vi "Update Library Icon.vi"(8 "error in (no error)":errorcluster, 11 "Mock Class Generator In":refnum<class "Responsive Mock Class Generator.lvclass">) -> (0 "error out":errorcluster, 3 "Mock Class Generator Out":refnum<class "Responsive Mock Class Generator.lvclass">)   [LabVIEW 2020, in "Responsive Mock Class Generator.lvclass"]
uses:
  Responsive Mock Class Generator.lvclass
  <vilib>/LabVIEW Icon API/lv_icon/Classes/Icon/Icon.lvclass
  <vilib>/LabVIEW Icon API/API_Rectangle Dimension.ctl
  <vilib>/LabVIEW Icon API/API_Text.ctl
  <vilib>/LabVIEW Icon API/API_Test Settings.ctl
  <vilib>/LabVIEW Icon API/lv_icon/Controls/Alignment.ctl
  <vilib>/LabVIEW Icon API/API_Text Colors.ctl
  <vilib>/LabVIEW Icon API/API_Rectangle Colors.ctl
  Responsive Mock Class Generator.lvclass/Responsive Mock Class Generator.ctl
  <vilib>/LabVIEW Icon API/LabVIEW Icon API.lvlib
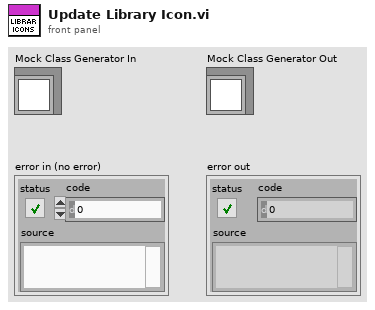
[diagram p1: front panel]
types:
  T1 = typedef "LabVIEW Icon API.lvlib/API_Rectangle Colors.ctl" = cluster{"Border":u32, "Background":u32}
  T2 = typedef "LabVIEW Icon API.lvlib/API_Test Settings.ctl" = cluster{"Font":string, "Alignment":T3, "Size":u8, "Center text":bool, "Capitalize text":bool, "Text color":T4}
  T3 = typedef "Alignment.ctl" = u16
  T4 = typedef "LabVIEW Icon API.lvlib/API_Text Colors.ctl" = cluster{"Line 1 color":u32, "Line 2 color":u32, "Line 3 color":u32, "Line 4 color":u32}
  T5 = typedef "LabVIEW Icon API.lvlib/API_Text.ctl" = cluster{"Line 1 text":string, "Line 2 text":string, "Line 3 text":string, "Line 4 text":string}
  T6 = typedef "LabVIEW Icon API.lvlib/API_Rectangle Dimension.ctl" = cluster{"Width":i16, "Height":i16}
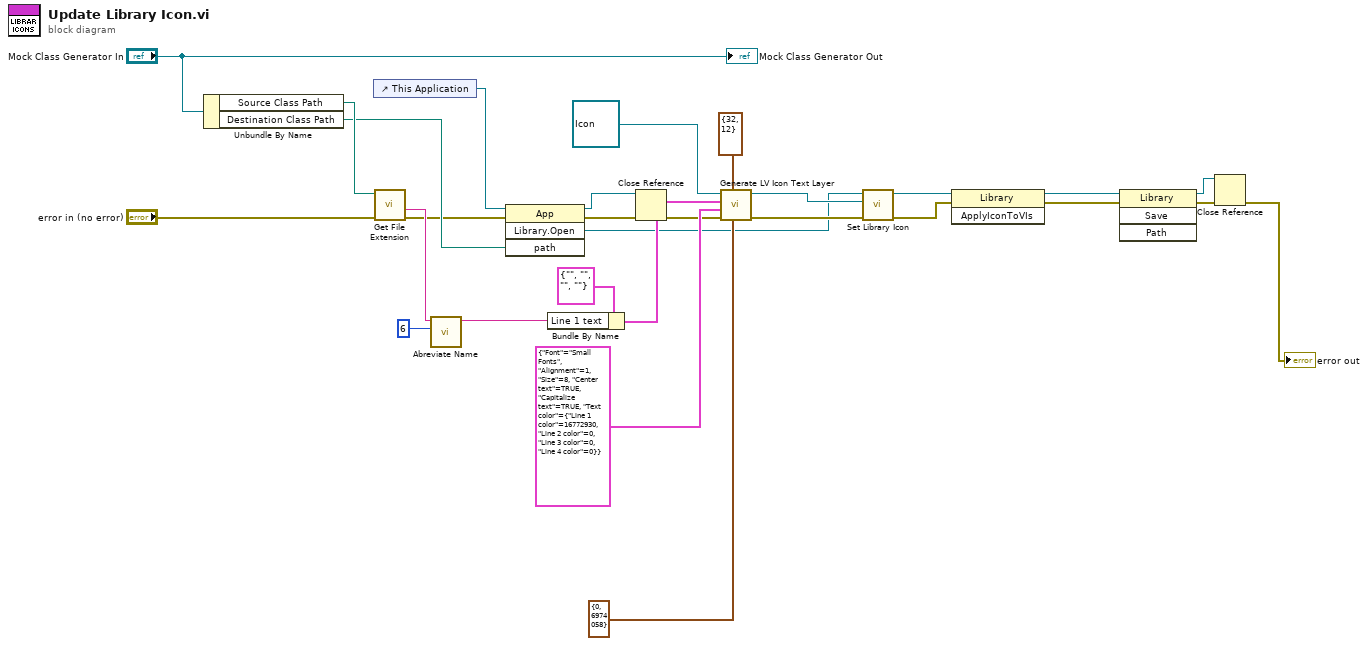
[diagram p0: block diagram]
diagram:
  n1 = Unbundle By Name("Mock Class Generator In") -> ("Source Class Path"=w21:path, "Destination Class Path"=w15:path)
  n2 = control-ref of="This Application"() -> (w16:refnum<vi>)
  n3 = call <vilib>:"Get File Extension.vi"("error in (no error)"="error in (no error)", "file"=w21) -> ("error out"=w11:errorcluster, "filename without extension"=w20:string)  [unwired: 5 in, 3 out]
  n4 = call "Abreviate Name.vi"("Max Length"=6, "Long Name in"=w20) -> ("Long Name out"=w17:string)  [unwired: 9 in]
  n5 = invoke class="App" method="Library.Open"(reference=w16, error in=w11, "path"=w15) -> (reference out=w1:refnum<vi>, error out=w10:errorcluster, "Open Library"=w9:refnum<vi>)  [unwired: 1 in, 1 out]
  n6 = Bundle By Name(cluster=T5 {"Line 1 text"="", "Line 2 text"="", "Line 3 text"="", "Line 4 text"=""} ("Text"), "Line 1 text"=w17) -> (w24:T5)
  n7 = Close Reference(reference=w1, error in (no error)=w10) -> (error out=w2:errorcluster)
  n8 = call <vilib>:"Generate LV Icon Text Layer.vi"("Rectangle colors (black, white)"=T1 {"Border"=0, "Background"=6974058}, "Rectangle dimension (32,32)"=T6 {"Width"=32, "Height"=12}, "error in (no error)"=w2, "Text settings"=T2 {"Font"="Small Fonts", "Alignment"=1, "Size"=8, "Center text"=TRUE, "Capitalize text"=TRUE, "Text color"={"Line 1 color"=16772930, "Line 2 color"=0, "Line 3 color"=0, "Line 4 color"=0}}, "Text"=w24, "Icon in"=refnum<class "Icon.lvclass"> refnum ("Icon.lvclass in")) -> ("error out"=w13:errorcluster, "Icon out"=w19:refnum<class "Icon.lvclass">)  [unwired: 4 in]
  n9 = call <vilib>:"Set Library Icon.vi"("error in (no error)"=w13, "Icon"=w19, "Library Refnum in"=w9) -> ("error out"=w12:errorcluster, "Library Refnum out"=w7:refnum<vi>)  [unwired: 7 in]
  n10 = invoke class="Library" method="ApplyIconToVIs"(reference=w7, error in=w12) -> (reference out=w4:refnum<vi>, error out=w8:errorcluster)  [unwired: 1 in, 1 out]
  n11 = invoke class="Library" method="Save"(reference=w4, error in=w8) -> (reference out=w3:refnum<vi>, error out=w6:errorcluster)  [unwired: 2 in, 2 out]
  n12 = Close Reference(reference=w3, error in (no error)=w6) -> (error out=→"error out":errorcluster)
  "Mock Class Generator Out" <- "Mock Class Generator In"
